vi "Create Configuration From File.vi"(8 "error in (no error)":errorcluster, 10 "Path in":path, 11 "Device Item Ref in":T1 format="%.0x") -> (0 "error out":errorcluster, 3 "Ref out":T1 format="%.0x")   [LabVIEW 2015, in "Instrument Addon System Explorer.lvlib"]
uses:
  Instrument Addon System Explorer.lvlib
  <vilib>/NI Veristand/Custom Device API/Custom Device Item Ref.ctl
  Export Import Utility/Instrument Custom Device SysDef Configuration V1.0.1.ctl
  Shared/Types/RSXXX Port Settings.ctl
  Export Import Utility/MetaData Channel Configuration.ctl
  Shared/Types/MetaData Parameters.ctl
  Shared/Types/Protocol Data Type.ctl
  Shared/Types/Metadata Channel Type.ctl
  Shared/Types/Type Cast Type.ctl
  Types/Channel Properties.ctl
  Export Import Utility/Message Group Configuration.ctl
  Export Import Utility/Message Configuration.ctl
  Export Import Utility/Command Message Configuration.ctl
  Shared/Types/Command Parameters.ctl
  Shared/Types/Linked Channel Cluster.ctl
  Export Import Utility/Response Message Configuration.ctl
  Shared/Types/Response Parameters.ctl
  Shared/Types/Response Wait Type.ctl
  Export Import Utility/Data Channel Configuration.ctl
  Shared/Types/Data Parameters.ctl
  Shared/Types/Data Channel Type.ctl
  Shared/Types/Message Parameters.ctl
  Shared/Types/Message Generation Type.ctl
  Shared/Types/Trigger Parameters.ctl
  Shared/Types/VISA Settings.ctl
  Shared/Types/TCPIP Settings.ctl
  Shared/Types/UDP Settings.ctl
  <vilib>/NI/GXML/_subVIs/GXML SearchParser/Search Parser.vi
  Shared/Instrument Addon Shared.lvlib
  <vilib>/NI/GXML/GXML.lvlib
  <vilib>/NI Veristand/Custom Device API/Custom Device API.lvlib
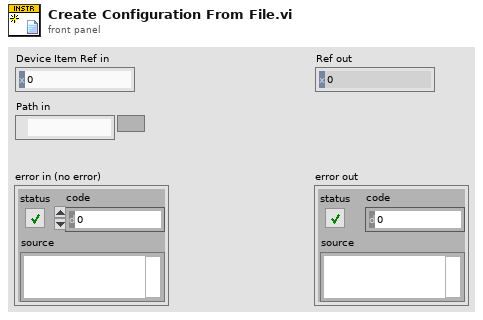
[diagram p1: front panel]
types:
  T1 = typedef "Custom Device API.lvlib/Custom Device Item Ref.ctl" = u64
  T2 = typedef "Instrument Addon System Explorer.lvlib/Instrument Custom Device SysDef Configuration V1.0.1.ctl" = cluster{"Name":string, "Description":string, "Protocol":string, "RS232 Config":T3, "MetaData Globals":T4[], "Message Groups":T10[], "GPIB Config":T24, "TCPIP Config":T25, "Decimation":u32, "UDP Config":T26}
  T3 = typedef "Instrument Addon Shared.lvlib/RSXXX Port Settings.ctl" = cluster{"Port":string, "Baud Rate":u32, "Data Bits":u16, "Parity":enum16{"None", "Odd", "Even", "Mark", "Space"}, "Stop Bits":u16, "Flow Control":u16, "XON":enum16{"NUL", "SOH", "STX", "ETX", "EOT", "ENQ", "ACK", "BEL", "BS", "HT", "LF", "VT", "FF", "CR", "SO", "SI", "DLE", "DC1", "DC2", "DC3", "DC4", "NAK", "SYN", "ETB", "CAN", "EM", "SUB", "ESC", "FS", "GS", "RS", "US", "SP", "!", "\"", "#", "$", "%", "&", "'", "(", ")", "*", "+", ",", "- (-)", ".", "/", "0", "1", "2", "3", "4", "5", "6", "7", "8", "9", ":", ";", "<", "=", ">", "?", "@", "A", "B", "C", "D", "E", "F", "G", "H", "I", "J", "K", "L", "M", "N", "O", "P", "Q", "R", "S", "T", "U", "V", "W", "X", "Y", "Z", "[", "\\", "]", "^", "_", "`", "a", "b", "c", "d", "e", "f", "g", "h", "i", "j", "k", "l", "m", "n", "o", "p", "q", "r", "s", "t", "u", "v", "w", "x", "y", "z", "{", "|", "}", "~"}, "XOFF":enum16{"NUL", "SOH", "STX", "ETX", "EOT", "ENQ", "ACK", "BEL", "BS", "HT", "LF", "VT", "FF", "CR", "SO", "SI", "DLE", "DC1", "DC2", "DC3", "DC4", "NAK", "SYN", "ETB", "CAN", "EM", "SUB", "ESC", "FS", "GS", "RS", "US", "SP", "!", "\"", "#", "$", "%", "&", "'", "(", ")", "*", "+", ",", "- (-)", ".", "/", "0", "1", "2", "3", "4", "5", "6", "7", "8", "9", ":", ";", "<", "=", ">", "?", "@", "A", "B", "C", "D", "E", "F", "G", "H", "I", "J", "K", "L", "M", "N", "O", "P", "Q", "R", "S", "T", "U", "V", "W", "X", "Y", "Z", "[", "\\", "]", "^", "_", "`", "a", "b", "c", "d", "e", "f", "g", "h", "i", "j", "k", "l", "m", "n", "o", "p", "q", "r", "s", "t", "u", "v", "w", "x", "y", "z", "{", "|", "}", "~"}, "End Read on Termination Character":bool, "End Write on Termination Character":bool, "Termination Character":u8}
  T4 = typedef "Instrument Addon System Explorer.lvlib/MetaData Channel Configuration.ctl" = cluster{"Name":string, "Description":string, "MetaData Parameters":T5, "Config GUID":string, "Channel Array":T9[]}
  T5 = typedef "Instrument Addon Shared.lvlib/MetaData Parameters.ctl" = cluster{"Data Type":T6, "Channel Type":T7, "List":string[], "Format String":string, "Type":T8, "Delimiter":string}
  T6 = typedef "Instrument Addon Shared.lvlib/Protocol Data Type.ctl" = enum16{"Single Channel", "Array"}
  T7 = typedef "Instrument Addon Shared.lvlib/Metadata Channel Type.ctl" = enum16{"Enumerated List", "Format", "Type Cast"}
  T8 = typedef "Instrument Addon Shared.lvlib/Type Cast Type.ctl" = enum16{"DBL", "SGL", "U64", "U32", "U16", "U8", "I64", "I32", "I16", "I8"}
  T9 = typedef "Instrument Addon System Explorer.lvlib/Channel Properties.ctl" = cluster{"Name":string, "Units":string, "Default Value":dbl}
  T10 = typedef "Instrument Addon System Explorer.lvlib/Message Group Configuration.ctl" = cluster{"Name":string, "Description":string, "Messages":T11[]}
  T11 = typedef "Instrument Addon System Explorer.lvlib/Message Configuration.ctl" = cluster{"Name":string, "Description":string, "Command":T12, "Response":T15, "Message Settings":T21, "Periodic Enabled":dbl, "Trigger Parameters":T23}
  T12 = typedef "Instrument Addon System Explorer.lvlib/Command Message Configuration.ctl" = cluster{"Description":string, "Command Parameters":T13, "MetaData Channels":T4[]}
  T13 = typedef "Instrument Addon Shared.lvlib/Command Parameters.ctl" = cluster{"Command":string, "Linked Channels":T14[], "Pad":bool, "Length":u32, "Pad Value":u8}
  T14 = typedef "Instrument Addon Shared.lvlib/Linked Channel Cluster.ctl" = cluster{"Variable Name":string, "GUID":string}
  T15 = typedef "Instrument Addon System Explorer.lvlib/Response Message Configuration.ctl" = cluster{"Description":string, "Reponse Parameters":T16, "Data Channels":T18[]}
  T16 = typedef "Instrument Addon Shared.lvlib/Response Parameters.ctl" = cluster{"Response":string, "Linked Channels":T14[], "Type Value":dbl, "Wait Type":T17, "Use Channel":bool, "Channel Path":string}
  T17 = typedef "Instrument Addon Shared.lvlib/Response Wait Type.ctl" = enum16{"Byte Count", "Wait sec"}
  T18 = typedef "Instrument Addon System Explorer.lvlib/Data Channel Configuration.ctl" = cluster{"Name":string, "Description":string, "Data Parameters":T19, "Config GUID":string, "Channel Array":T9[]}
  T19 = typedef "Instrument Addon Shared.lvlib/Data Parameters.ctl" = cluster{"Data Type":T6, "Channel Type":T20, "Format String":string, "Expected String":string, "Type":T8, "List":string[], "Delimiter":string}
  T20 = typedef "Instrument Addon Shared.lvlib/Data Channel Type.ctl" = enum16{"Format", "Comparison", "Type Cast", "Enumerated List"}
  T21 = typedef "Instrument Addon Shared.lvlib/Message Parameters.ctl" = cluster{"Generation Type":T22, "Period":dbl, "Include Protection":bool, "Type":string}
  T22 = typedef "Instrument Addon Shared.lvlib/Message Generation Type.ctl" = enum16{"Trigger Only", "Periodic & Trigger"}
  T23 = typedef "Instrument Addon Shared.lvlib/Trigger Parameters.ctl" = cluster{"Use Channel":bool, "Channel Path":string}
  T24 = typedef "Instrument Addon Shared.lvlib/VISA Settings.ctl" = cluster{"VISA Resource":string, "Enable Termination Character":bool, "Termination Character":u8, "Timeout":u32, "Append Write Termination Character":bool}
  T25 = typedef "Instrument Addon Shared.lvlib/TCPIP Settings.ctl" = cluster{"IP Address":string, "Port":u16}
  T26 = typedef "Instrument Addon Shared.lvlib/UDP Settings.ctl" = cluster{"Local IP Address":string, "Local Port":u16, "Target IP Address":string, "Target Port":u16}
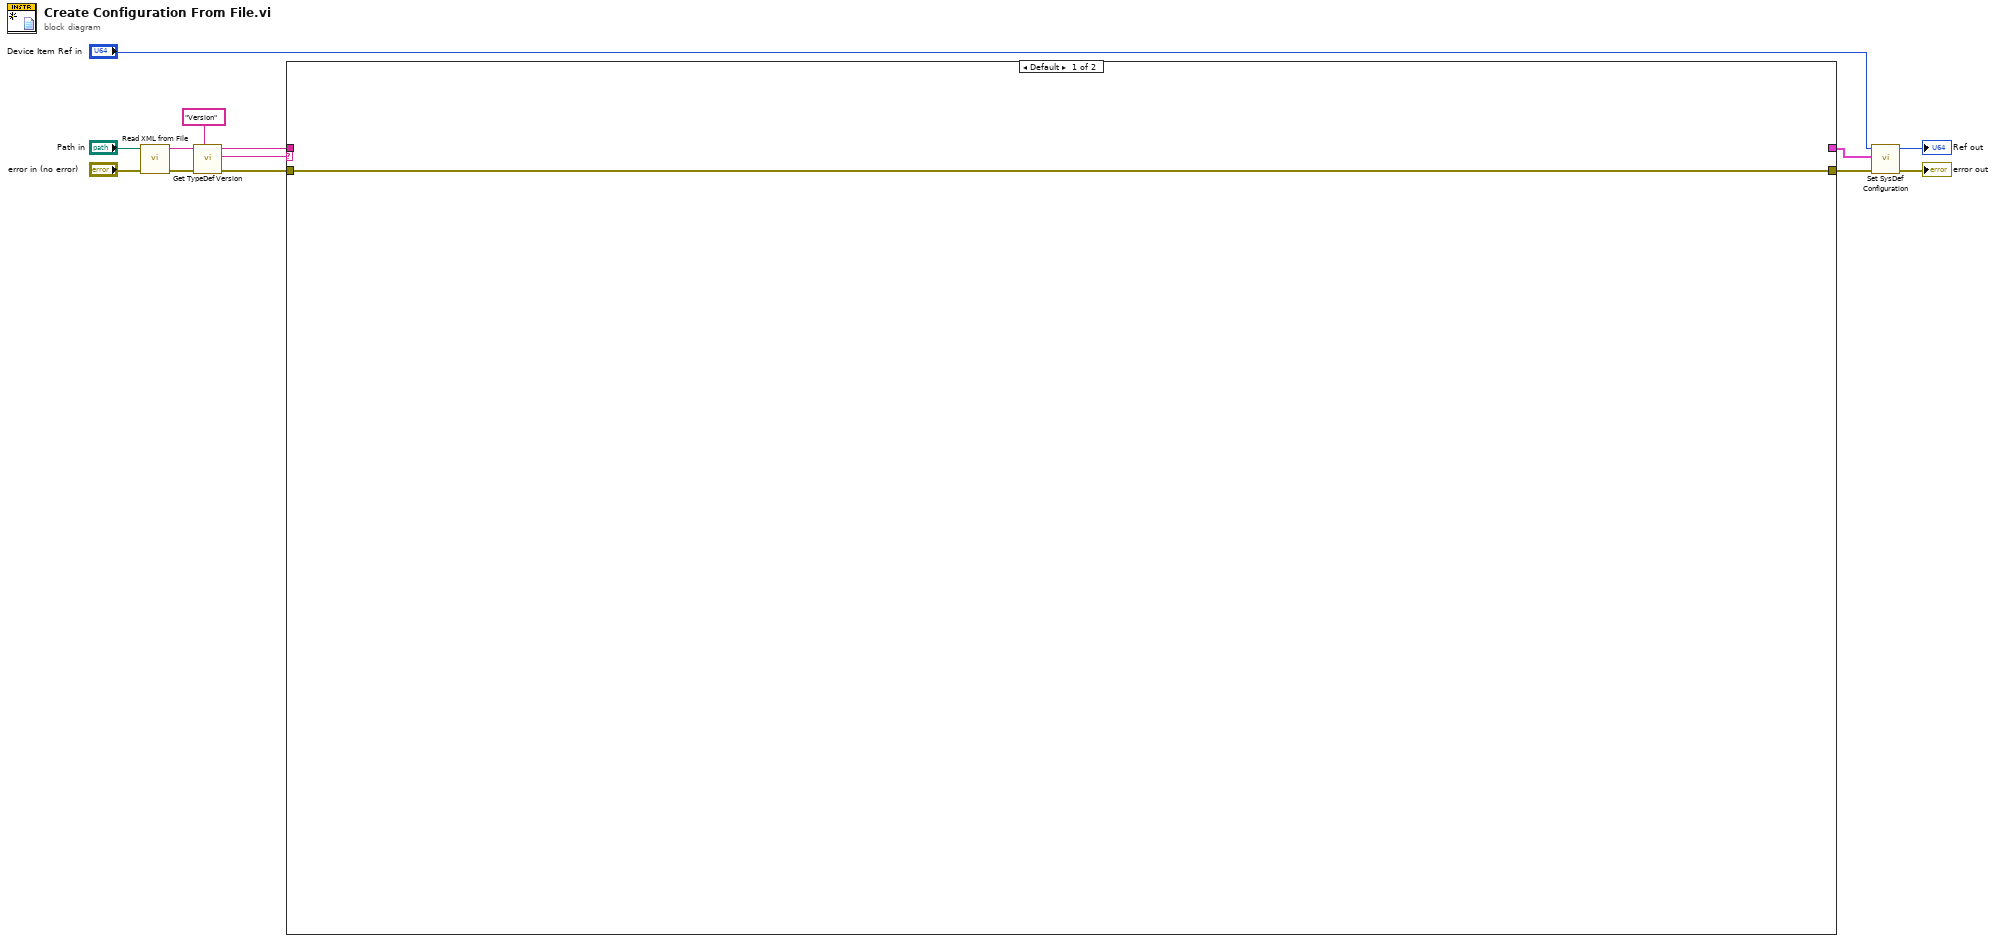
[diagram p0: block diagram]
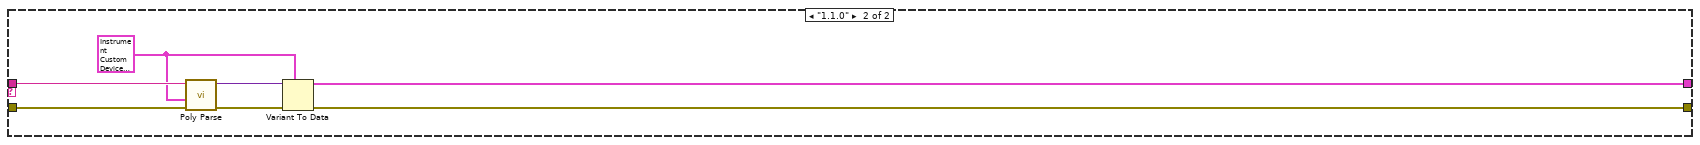
[diagram p2: hidden frame]
diagram:
  n1 = call <vilib>:"Read XML from File.vi"("error in"="error in (no error)", "XML File Path"="Path in") -> ("error out"=w11:errorcluster, "XML String Out"=w10:string)  [unwired: 8 in]
  n2 = call <vilib>:"Get TypeDef Version.vi"("Version Tag Name"="Version", "error in"=w11, "XML String In"=w10) -> ("error out"=w7:errorcluster, "Version String"=w6:string, "XML String Out"=w8:string)  [unwired: 6 in]
  n3 = case shown="Default" w6 {
    tunnel: w8 -> [_ w21]
    tunnel: w7 -> [w14 w20]
    tunnel: [_ w15] -> w3
    tunnel: [w14 w17] -> w1
    frame Default {
    }
    frame "1.1.0" {
      w16 = T2 {"Name"="", "Description"="", "Protocol"="", "RS232 Config"={"Port"="", "Baud Rate"=0, "Data Bits"=0, "Parity"=enum."None", "Stop Bits"=0, "Flow Control"=0, "XON"=enum."NUL", "XOFF"=enum."NUL", "End Read on Termination Character"=FALSE, "End Write on Termination Character"=FALSE, "Termination Character"=0}, "MetaData Globals"=[], "Message Groups"=[], "GPIB Config"={"VISA Resource"="", "Enable Termination Character"=FALSE, "Termination Character"=0, "Timeout"=0, "Append Write Termination Character"=FALSE}, "TCPIP Config"={"IP Address"="", "Port"=0}, "Decimation"=0, "UDP Config"={"Local IP Address"="", "Local Port"=0, "Target IP Address"="", "Target Port"=0}} ("Configuration")
      n4 = call-poly <vilib>:"Poly Parse.vi"("error in"=w20, "TypeDesc"=w16, "XML String In"=w21) -> ("error out"=w19:errorcluster, "Parsed Data"=w18:variant)  [unwired: 7 in]
      n5 = Variant To Data(error in=w19, type=w16, Variant=w18) -> (data=w15:T2, error out=w17:errorcluster)
    }
  }
  n6 = call "Set SysDef Configuration.vi"("error in (no error)"=w1, "Configuration"=w3, "Node Ptr"="Device Item Ref in") -> ("error out"=→"error out":errorcluster, "Ref out"=→"Ref out":T1)  [unwired: 7 in]
